vi "Parse HTTP Response.vi"(11 "HTTP Response":string) -> (0 "Body":string, 1 "Header":string, 2 "Status":string, 3 "Location":string, 5 "HTTP Version":string, 7 "Method":string)   [LabVIEW 2020]
uses:
  <vilib>/regexp/Match Regular Expression.xnode
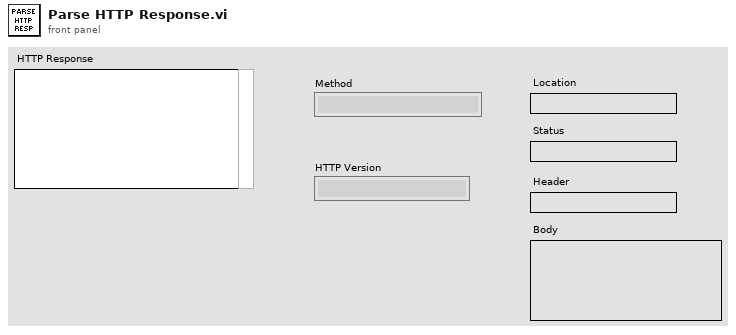
[diagram p1: front panel]
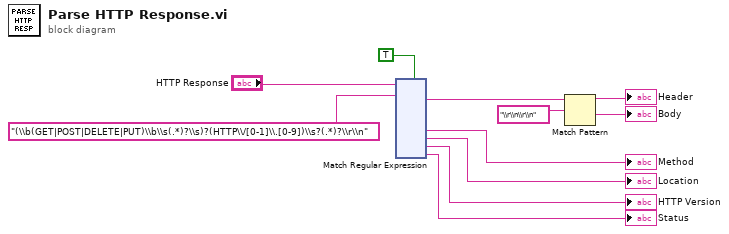
[diagram p0: block diagram]
diagram:
  n1 = xnode "Match Regular Expression"("input string"="HTTP Response", "regular expression"="(\\b(GET|POST|DELETE|PUT)\\b\\s(.*)?\\s)?(HTTP\\/[0-1]\\.[0-9])\\s?(.*)?\\r\\n", "multiline? (F)"=TRUE) -> ("after match"=w8:string, "submatch 2"=→"Method":string, "submatch 3"=→"Location":string, "submatch 4"=→"HTTP Version":string, "submatch 5"=→"Status":string)  [unwired: 3 in, 5 out]
  n2 = Match Pattern(string=w8, regular expression="\\r\\n\\r\\n") -> (before substring=→"Header":string, after substring=→"Body":string)  [unwired: 1 in, 2 out]
